vi "Host.vi"() -> ()   [LabVIEW 2025]
uses:
  <vilib>/rvi/interface/nirviOpenFPGA/nirviOpenFPGA.xnode
  <vilib>/rvi/interface/nirviMethod/nirviMethod.xnode
  <vilib>/FPGAPlugInAG/Dynamic/niLvFpga_WriteFifo_Dynamic.vi
  <vilib>/rvi/errors/niLvFpgaMergeErrorWithErrorCode.vi
  <vilib>/FPGAPlugInAG/Dynamic/niLvFpga_Run_Dynamic.vi
  <vilib>/FPGAPlugInAG/Dynamic/niLvFpga_Reset_Dynamic.vi
  <vilib>/rvi/interface/nirviCloseFPGA/nirviCloseFPGA.xnode
  <vilib>/FPGAPlugInAG/Dynamic/niLvFpga_ReadFifo_Dynamic.vi
  <vilib>/FPGAPlugInAG/Dynamic/niLvFpga_Close_Dynamic.vi
  FPGA Bitfiles/hmmlponfpga_FPGATarget_Target_Y6+8hyRHR-w.lvbitx
  Target.vi
  <vilib>/FPGAPlugInAG/cRIO-9035/niLvFpga_Open_cRIO-9035.vi
  <vilib>/rvi/interface/common/dynamic/niFpgaDynamicAddResources.vi
panel:
  out "Uncontrolled Acceleration":dynamicdata(graph)
  out "Uncontrolled Velocity":dynamicdata(graph)
  out "Control Force":sgl[](graph)
  out "Uncontrolled Displacement":dynamicdata(graph)
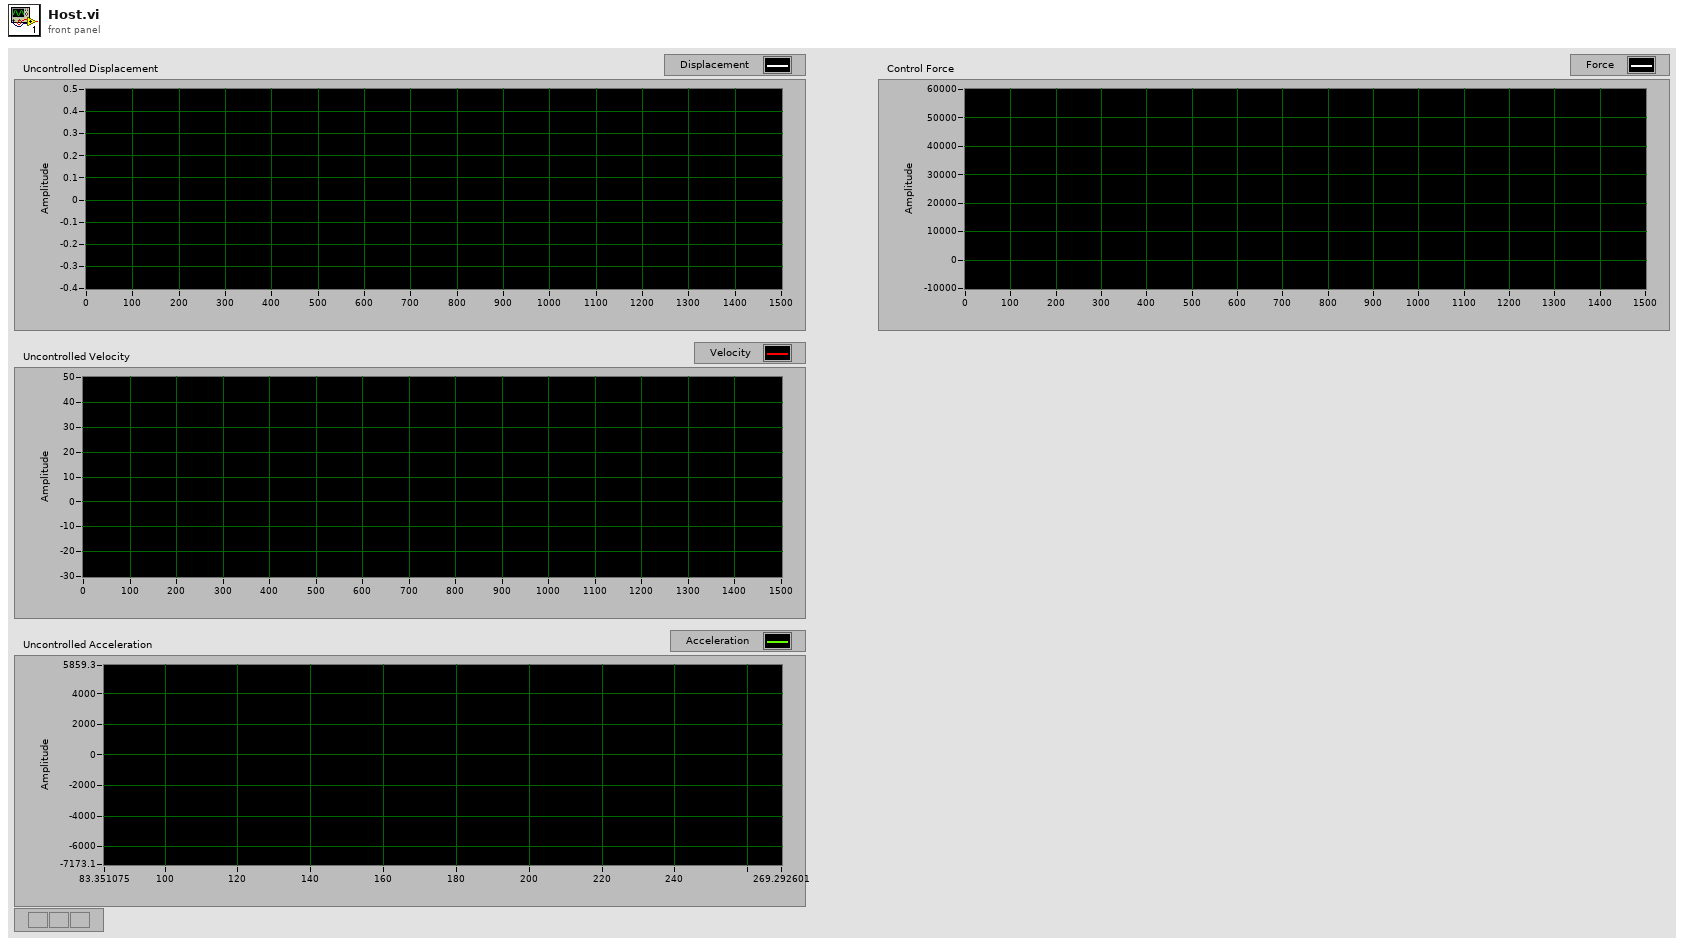
[diagram p1: front panel]
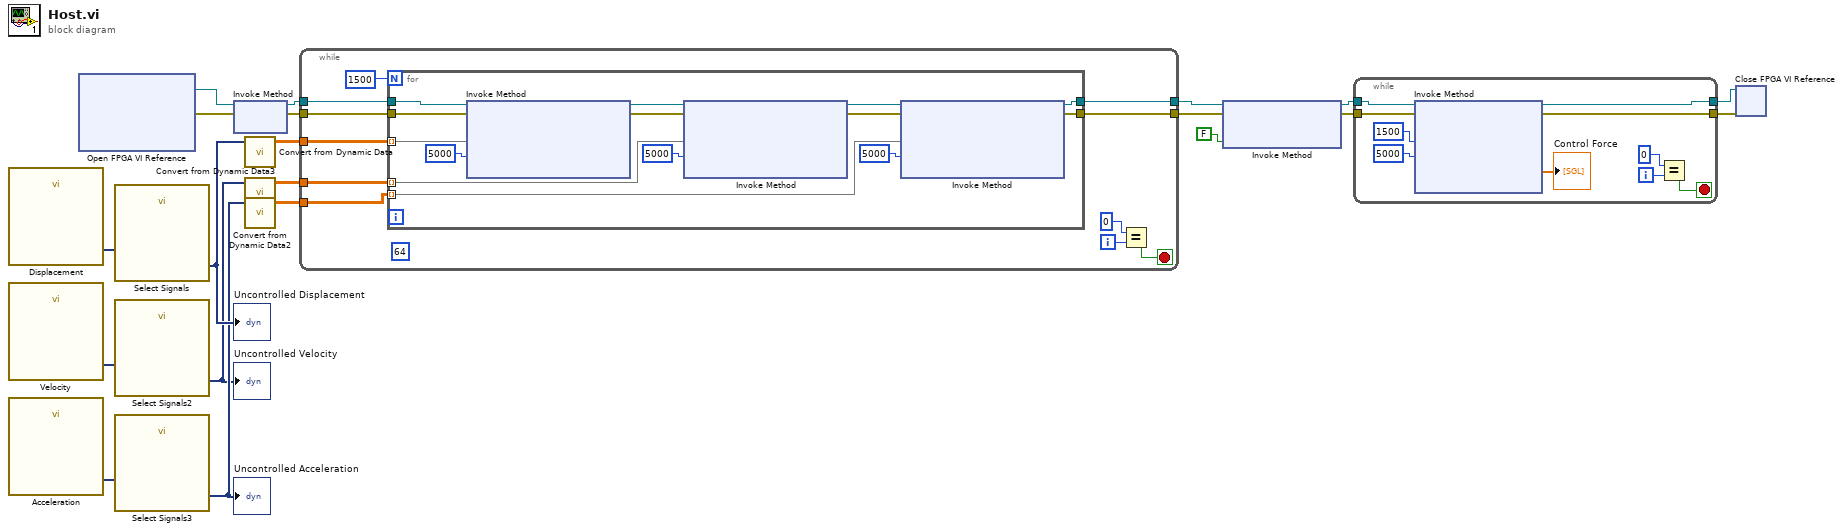
[diagram p0: block diagram]
diagram:
  n1 = call "Displacement"() -> ("Signals"=w17:dynamicdata)  [unwired: 6 in, 5 out]
  n2 = call "Velocity"() -> ("Signals"=w20:dynamicdata)  [unwired: 6 in, 5 out]
  n3 = call "Acceleration"() -> ("Signals"=w19:dynamicdata)  [unwired: 6 in, 5 out]
  n4 = xnode "Open FPGA VI Reference"() -> ("FPGA VI Reference Out"=w18:refnum<k20>, "error out"=w8:errorcluster)  [unwired: 2 in]
  n5 = call "Select Signals"("Signals"=w17) -> ("Signal Out"=w5:dynamicdata)  [unwired: 9 in, 1 out]
  "Uncontrolled Displacement" <- w5
  n6 = call "Select Signals2"("Signals"=w20) -> ("Signal Out"=w3:dynamicdata)  [unwired: 9 in, 1 out]
  "Uncontrolled Velocity" <- w3
  n7 = call "Select Signals3"("Signals"=w19) -> ("Signal Out"=w4:dynamicdata)  [unwired: 9 in, 1 out]
  "Uncontrolled Acceleration" <- w4
  n8 = xnode "Invoke Method"("FPGA VI Reference In"=w18, "error in"=w8) -> ("FPGA VI Reference Out"=w10:refnum<k20>, "error out"=w9:errorcluster)
  n9 = call "Convert from Dynamic Data"("Dynamic Data Type"=w5) -> ("Array"=w13:dbl[][])  [unwired: 3 in]
  n10 = call "Convert from Dynamic Data3"("Dynamic Data Type"=w3) -> ("Array"=w11:dbl[][])  [unwired: 3 in]
  n11 = call "Convert from Dynamic Data2"("Dynamic Data Type"=w4) -> ("Array"=w12:dbl[][])  [unwired: 3 in]
  n12 = while {
    tunnel: w10 -> [w31]
    tunnel: w9 -> [w29]
    tunnel: w11 -> [w28]
    tunnel: w12 -> [w27]
    tunnel: w13 -> [w23]
    tunnel: [w22] -> w2
    tunnel: [w21] -> w1
    i -> [w26]
    stop <- w24 stop-if-true
    (unwired) 64
    n13 = for {
      N: 1500 -> [_]
      tunnel: w31 -> [w45]
      tunnel: w29 -> [w42]
      tunnel: [w39] -> w22
      tunnel: [w38] -> w21
      tunnel: w28 -> [w36] mode=indexing
      tunnel: w27 -> [w32] mode=indexing
      tunnel: w23 -> [w37] mode=indexing
      n14 = xnode "Invoke Method"("FPGA VI Reference In"=w45, "error in"=w42, "Data"=w37, "Timeout (ms)"=5000) -> ("FPGA VI Reference Out"=w44:refnum<k20>, "error out"=w43:errorcluster)  [unwired: 1 out]
      n15 = xnode "Invoke Method"("FPGA VI Reference In"=w44, "error in"=w43, "Data"=w36, "Timeout (ms)"=5000) -> ("FPGA VI Reference Out"=w40:refnum<k20>, "error out"=w41:errorcluster)  [unwired: 1 out]
      n16 = xnode "Invoke Method"("FPGA VI Reference In"=w40, "error in"=w41, "Data"=w32, "Timeout (ms)"=5000) -> ("FPGA VI Reference Out"=w39:refnum<k20>, "error out"=w38:errorcluster)  [unwired: 1 out]
    }
    n17 = Equal?(x=0, y=w26) -> (x = y?=w24:bool)
  }
  n18 = xnode "Invoke Method"("FPGA VI Reference In"=w2, "error in"=w1, "Wait Until Done (F)"=FALSE) -> ("FPGA VI Reference Out"=w15:refnum<k20>, "error out"=w14:errorcluster)
  n19 = while {
    tunnel: w15 -> [w55]
    tunnel: [w52] -> w7
    tunnel: w14 -> [w54]
    tunnel: [w53] -> w6
    i -> [w49]
    stop <- w50 stop-if-true
    n20 = xnode "Invoke Method"("FPGA VI Reference In"=w55, "error in"=w54, "Number of Elements"=u32 1500, "Timeout (ms)"=5000) -> ("FPGA VI Reference Out"=w52:refnum<k20>, "error out"=w53:errorcluster, "Data"=→"Control Force":sgl[])  [unwired: 1 out]
    n21 = Equal?(x=0, y=w49) -> (x = y?=w50:bool)
  }
  n22 = xnode "Close FPGA VI Reference"("FPGA VI Reference In"=w7, "error in"=w6) -> ()  [unwired: 1 out]
